vi "Channel Info.vi"(8 "error in":errorcluster, 11 "Plugin_Channels in":refnum<class "Plugin_Channels.lvclass">) -> (0 "error out":errorcluster, 1 "Channel Active?":bool, 2 "Channel Information":T1={"Channel Direction"=enum."Module Output", "Alias"="", "Refresh (ms)"=1000.0, "Scaling Information"={"Active"=FALSE, "Scaling Type"=enum."Linear", "Output Minimum"=0.0, "Output Maximum"=1.0, "Raw Minimum"=0.0, "Raw Maximum"=1.0, "Output Unit"="", "Function"="", "Lookup Table"=""}, "Value Type"=enum."double", "Subchannels"=[], "Auxiliary Data"=variant, "Group"=-1}, 3 "Plugin_Channels out":refnum<class "Plugin_Channels.lvclass">)   [LabVIEW 2020, in "Plugin.lvlib" / "Plugin_Channels.lvclass"]
doc: "Update Channel Information VI of the Parent Channel class."
uses:
  Plugin_Channels.lvclass
  builds/Libraries/LabSys Framework.lvlibp/Configuration Storage/Test Configuration/Channel Information.ctl
  builds/Libraries/LabSys Framework.lvlibp/Configuration Storage/Test Configuration/Channel Directions.ctl
  builds/Libraries/LabSys Framework.lvlibp/Configuration Storage/Test Configuration/Scaling Information.ctl
  builds/Libraries/LabSys Framework.lvlibp/Configuration Storage/Test Configuration/Scaling Types.ctl
  builds/Libraries/Framework Base Library.lvlibp/Value Types.ctl
  builds/Libraries/LabSys Framework.lvlibp/Configuration Storage/Test Configuration/Subchannel Information.ctl
  builds/Libraries/Framework Base Library.lvlibp
  builds/Libraries/LabSys Framework.lvlibp/Configuration Storage/Test Configuration/Test Configuration.lvclass
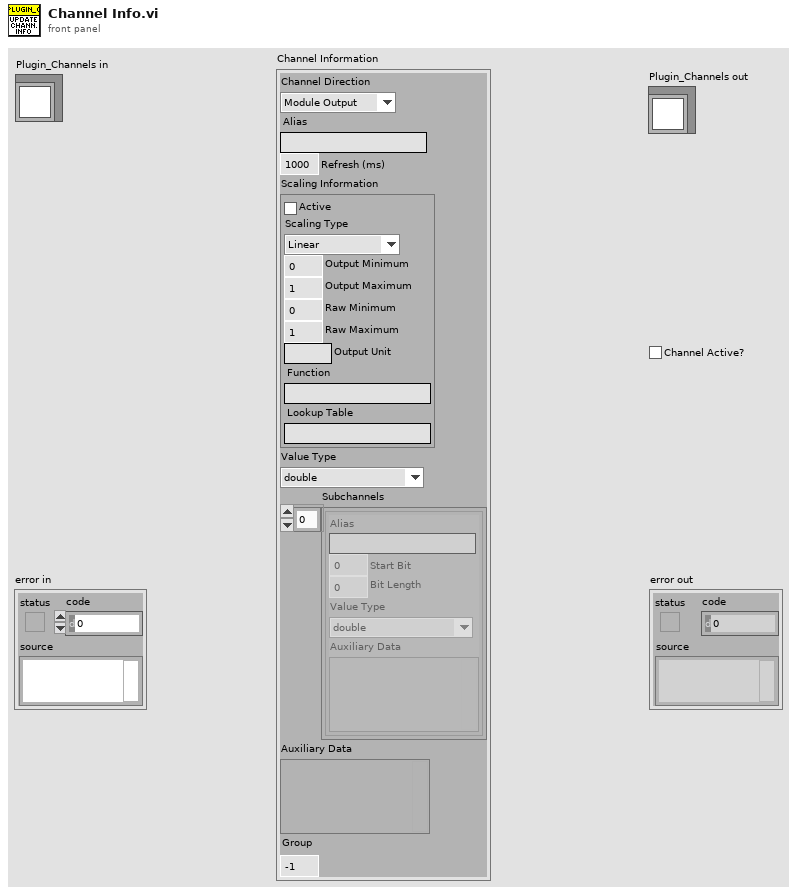
[diagram p1: front panel]
types:
  T1 = typedef "LabSys Framework.lvlibp/Configuration Storage.lvlib/Test Configuration.lvclass/Channel Information.ctl" = cluster{"Channel Direction":T2, "Alias":string, "Refresh (ms)":dbl, "Scaling Information":T3, "Value Type":T5, "Subchannels":T6[], "Auxiliary Data":variant, "Group":i32}
  T2 = typedef "LabSys Framework.lvlibp/Configuration Storage.lvlib/Test Configuration.lvclass/Channel Directions.ctl" = enum8{"Module Input", "Module Output"}
  T3 = typedef "LabSys Framework.lvlibp/Configuration Storage.lvlib/Test Configuration.lvclass/Scaling Information.ctl" = cluster{"Active":bool, "Scaling Type":T4, "Output Minimum":dbl, "Output Maximum":dbl, "Raw Minimum":dbl, "Raw Maximum":dbl, "Output Unit":string, "Function":string, "Lookup Table":string}
  T4 = typedef "LabSys Framework.lvlibp/Configuration Storage.lvlib/Test Configuration.lvclass/Scaling Types.ctl" = enum8{"Linear", "Function", "Lookup Table"}
  T5 = typedef "Framework Base Library.lvlibp/Value Types.ctl" = enum8{"Unknown", "double", "double array", "Waveform", "DigWaveform", "Boolean", "Decimal", "String", "Db2Message", "Byte Array", "Unsigned Decimal"}
  T6 = typedef "LabSys Framework.lvlibp/Configuration Storage.lvlib/Test Configuration.lvclass/Subchannel Information.ctl" = cluster{"Alias":string, "Start Bit":u32, "Bit Length":u32, "Value Type":T5, "Auxiliary Data":variant}
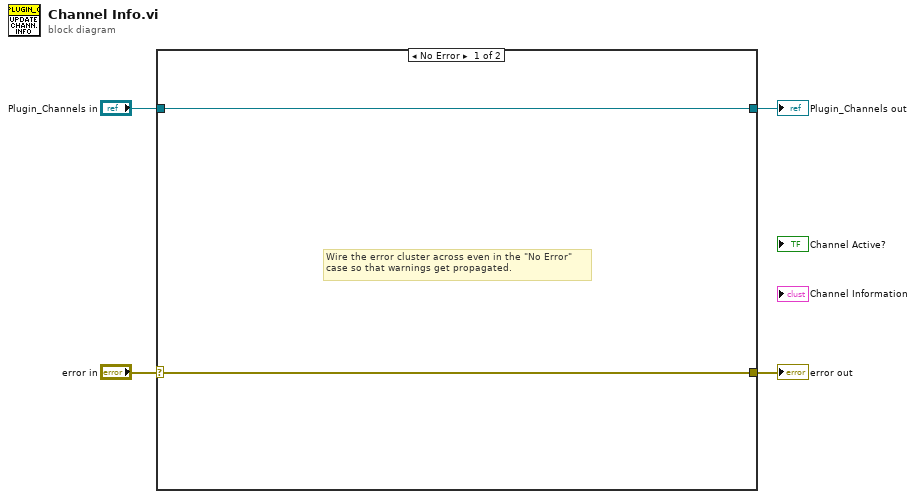
[diagram p0: block diagram]
diagram:
  n1 = case shown="No Error" "error in" {
    selector: "error in" -> [w5 w8]
    tunnel: [w5 w8] -> w3
    tunnel: [w6 w7] -> w1
    tunnel: "Plugin_Channels in" -> [w6 w7]
    frame No Error {
      # "Wire the error cluster across even in the \"No Error\"\ncase so that warnings get propagated."
    }
    frame Error {
    }
  }
  "error out" <- w3
  "Plugin_Channels out" <- w1
